vi "readMATFIle.vi"() -> ()   [LabVIEW 2024]
panel:
  out "substring before match":string
  out "offset past match":i32
  out "Waveform Graph":dbl[][](graph)
  out "extra":string
  out "BE":u32
  out "# bytes":u32
  out "data type":u32
  out "unknown":string
  out "name":string
  out "subsys data stuff":string
  out "value":dbl[](array[numeric]) format="%.6f"
  out "Endian indicator":string
  out "version":u16 format="%.0x"
  out "Title":string
  out "data":string
  # "16384"
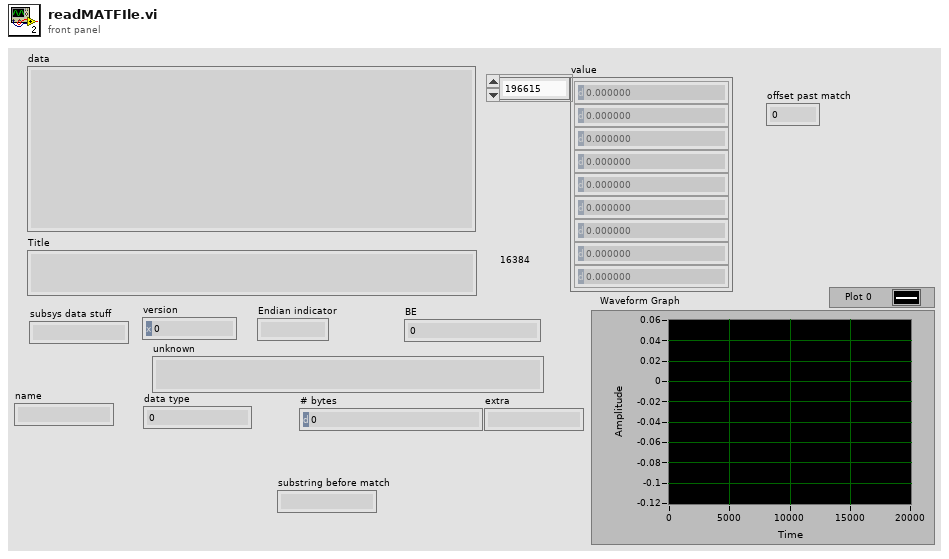
[diagram p1: front panel]
types:
  T1 = enum16{"big-endian, network order", "native, host order", "little-endian"}
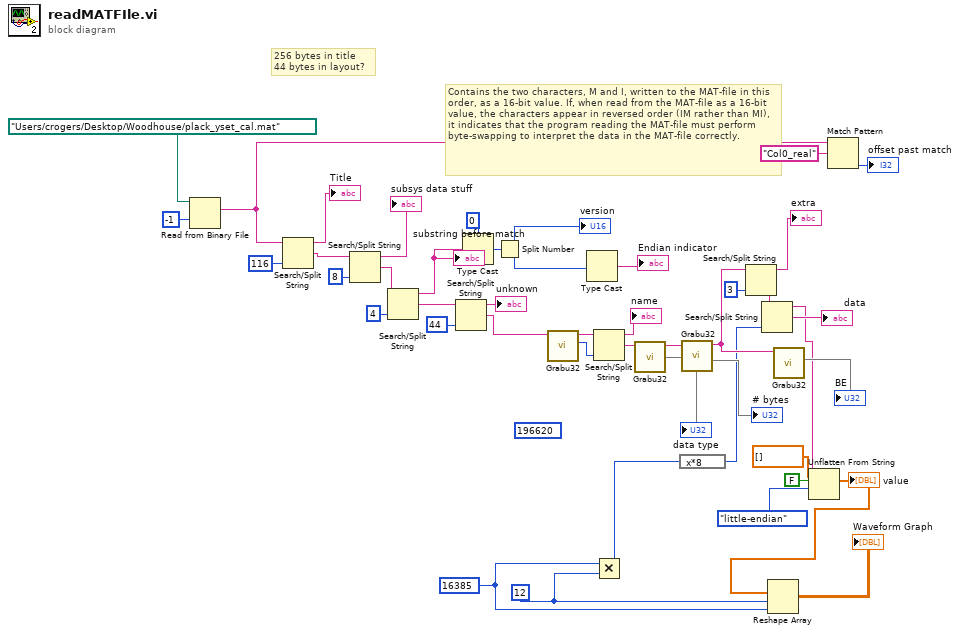
[diagram p0: block diagram]
diagram:
  w8 = 12 ("dimension size")
  w3 = 16385 ("dimension size")
  (unwired) 196620 ("offset (0)")
  # "Contains the two characters, M and I, written to the MAT-file in this order, as a 16-bit value. If, when read from the MAT-file as a 16-bit value, the characters appear in reversed order (IM rather than MI), it indicates that the program reading the MAT-file must perform byte-swapping to interpret the data in the MAT-file correctly."
  # "256 bytes in title\n44 bytes in layout?"
  n1 = Read from Binary File(10:-1 ("count (1)"), 11:path "/Users/crogers/Desktop/Woodhouse/plack_yset_cal.mat" ("file (use dialog)")) -> (2:w4:string)  [unwired: 4 in, 3 out]
  n2 = Search/Split String(string=w4, offset (0)=116) -> (substring before match=→"Title":string, match + rest of string=w42:string)  [unwired: 1 in, 1 out]
  n3 = Search/Split String(string=w42, offset (0)=8) -> (substring before match=→"subsys data stuff":string, match + rest of string=w39:string)  [unwired: 1 in, 1 out]
  n4 = Search/Split String(string=w39, offset (0)=4) -> (substring before match=w36:string, match + rest of string=w30:string)  [unwired: 1 in, 1 out]
  "substring before match" <- w36
  n5 = Search/Split String(string=w30, offset (0)=44) -> (substring before match=→"unknown":string, match + rest of string=w29:string)  [unwired: 1 in, 1 out]
  n6 = Type Cast(type=u32 0 ("offset (0)"), x=w36) -> (*(type *) &x=w35:u32)
  n7 = Split Number(x=w35) -> (hi(x)=→"version":u16, lo(x)=w2:u16)
  n8 = call "Grabu32.vi"("String in"=w29) -> ("Value"=w27:u32, "String out"=w28:string)  [unwired: 9 in]
  n9 = Type Cast(x=w2) -> (*(type *) &x=→"Endian indicator":string)  [unwired: 1 in]
  n10 = Search/Split String(string=w28, offset (0)=w27) -> (substring before match=→"name":string, match + rest of string=w24:string)  [unwired: 1 in, 1 out]
  n11 = Multiply(x=w3, y=w8) -> (x*y=w9:i32)
  n12 = call "Grabu32.vi"("String in"=w24) -> (1:→"data type", "String out"=w18:string)  [unwired: 8 in, 1 out]
  n13 = expression code="x*8"(w9) -> (w12:i32)
  n14 = call "Grabu32.vi"("String in"=w18) -> (1:→"# bytes", "String out"=w17:string)  [unwired: 8 in, 1 out]
  n15 = Search/Split String(string=w17, offset (0)=3) -> (substring before match=→"extra":string, match + rest of string=w14:string)  [unwired: 1 in, 1 out]
  n16 = Search/Split String(string=w14, offset (0)=w12) -> (substring before match=w7:string, match + rest of string=→"data":string)  [unwired: 1 in, 1 out]
  n17 = call "Grabu32.vi"("String in"=w17) -> (1:→"BE")  [unwired: 8 in, 2 out]
  n18 = Unflatten From String(type=dbl[] [], binary string=w7, data includes array or string size? (T)=FALSE, byte order (0:big-endian, network order)=T1."little-endian") -> (value=w11:dbl[])  [unwired: 1 in, 2 out]
  "value" <- w11
  n19 = Reshape Array(w11, w8, w3) -> (→"Waveform Graph":dbl[][])
  n20 = Match Pattern(string=w4, regular expression="Col0_real") -> (offset past match=→"offset past match":i32)  [unwired: 1 in, 3 out]
